vi "End Switch to Corridor.vi"(8 "Command Info In":T2, 10 "Block Inputs":T1, 11 "Starting Position":T5) -> (0 "Command Info Out":T2)   [LabVIEW 2017]
uses:
  <vilib>/Rock Robotics/WPI/Framework/Command Status Info.ctl
  <vilib>/Rock Robotics/WPI/Framework/Completion Status.ctl
  <vilib>/Rock Robotics/WPI/Framework/Completion Notifier.ctl
  Support Code/Starting Position.ctl
  Support Code/Extended Block Inputs.ctl
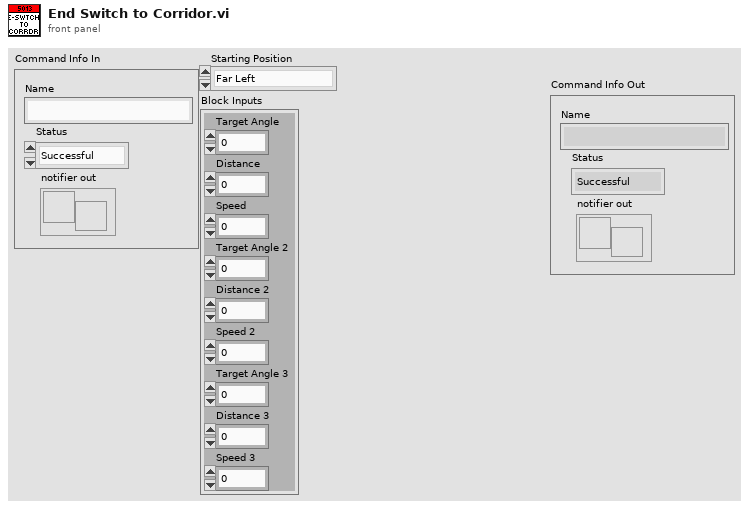
[diagram p1: front panel]
types:
  T1 = typedef "Extended Block Inputs.ctl" = cluster{"Target Angle":dbl, "Distance":dbl, "Speed":dbl, "Target Angle 2":dbl, "Distance 2":dbl, "Speed 2":dbl, "Target Angle 3":dbl, "Distance 3":dbl, "Speed 3":dbl}
  T2 = typedef "Command Status Info.ctl" = cluster{"Name":string, "Status":T3, "notifier out":T4}
  T3 = typedef "Completion Status.ctl" = enum16{"Successful", "Aborted", "Incomplete"}
  T4 = typedef "Completion Notifier.ctl" = refnum<notifier>
  T5 = typedef "Starting Position.ctl" = enum16{"Far Left", "Center", "Far Right"}
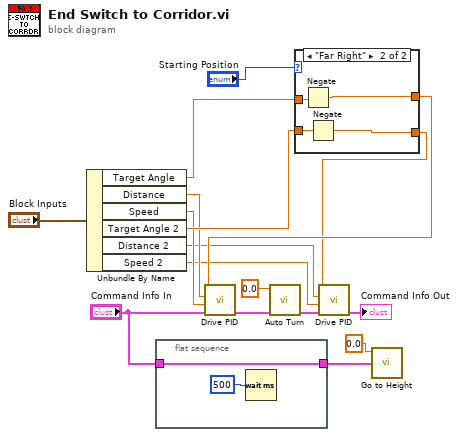
[diagram p0: block diagram]
diagram:
  n1 = Unbundle By Name("Block Inputs") -> ("Target Angle"=w7:dbl, "Distance"=w4:dbl, "Speed"=w3:dbl, "Target Angle 2"=w6:dbl, "Distance 2"=w2:dbl, "Speed 2"=w1:dbl)
  n2 = flat-sequence {
    tunnel: "Command Info In" -> [w18]
    tunnel: [w18] -> w10
    frame #0 {
      n3 = Wait (ms)(milliseconds to wait=u32 500 ("millisecond timer value")) -> ()  [unwired: 1 out]
    }
  }
  n4 = case shown="\"Far Right\"" "Starting Position" {
    tunnel: [w21 w25] -> w9
    tunnel: w7 -> [w21 w23]
    tunnel: w6 -> [w20 w24]
    tunnel: [w20 w22] -> w5
    frame "Far Left", Default {
    }
    frame "Far Right" {
      n5 = Negate(x=w23) -> (-x=w25:dbl)
      n6 = Negate(x=w24) -> (-x=w22:dbl)
    }
  }
  n7 = call "Drive PID.vi"("Command Info In"="Command Info In", "Speed"=w3, "Distance"=w4, "Target Angle"=w9) -> ("Command Info Out"=w16:T2)  [unwired: 7 in]
  n8 = call "Auto Turn.vi"("Command Info In"=w16, "Target Angle"=0.0) -> ("Command Info Out"=w15:T2)  [unwired: 9 in]
  n9 = call "Drive PID.vi"("Command Info In"=w15, "Speed"=w1, "Distance"=w2, "Target Angle"=w5) -> ("Command Info Out"=→"Command Info Out":T2)  [unwired: 7 in]
  n10 = call "Go to Height.vi"("Command Info In"=w10, "Target Height (in)"=0.0) -> ()  [unwired: 9 in, 1 out]
